vi "KalibrierInfoMessages.vi"(8 "Fehler (Eingang, kein Fehler)":errorcluster, 11 "Kalibrier Info-Cluster in":T1) -> (0 "error out":errorcluster, 3 "Kalibrier Info Messages Array":cluster{"Label.Text":string, "Wert":bool}[](array[cluster]))   [LabVIEW 2020, in "Linearisierung v2.lvlib" / "SpanEinstellungen.lvlib"]
uses:
  SpanEinstellungen.lvlib
  Kalibrier Info Cluster.ctl
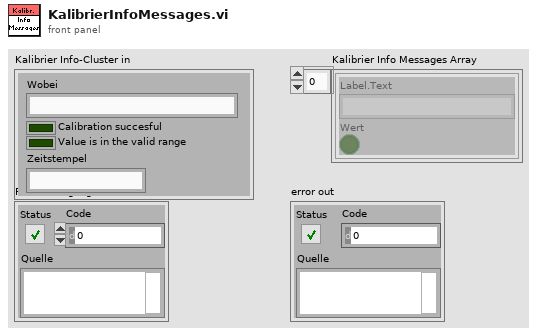
[diagram p1: front panel]
types:
  T1 = typedef "Linearisierung v2.lvlib/SpanEinstellungen.lvlib/Kalibrier Info Cluster.ctl" = cluster{"Wobei":string, "Calibration succesful":bool, "Value is in the valid range":bool, "Zeitstempel":string}
  T2 = cluster{bool, "Calibration succesful":bool, "Value is in the valid range":bool}
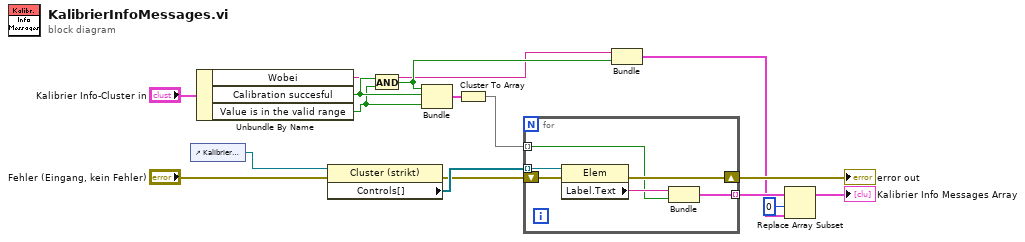
[diagram p0: block diagram]
diagram:
  n1 = control-ref of="Kalibrier Info-Cluster in"() -> (w8:refnum<vi>)
  n2 = Unbundle By Name("Kalibrier Info-Cluster in") -> ("Wobei"=w1:string, "Calibration succesful"=w7:bool, "Value is in the valid range"=w6:bool)
  n3 = property class="Cluster (strikt)"(reference=w8, error in="Fehler (Eingang, kein Fehler)") -> (error out=w14:errorcluster, "Controls[]"=w16:refnum<vi>[])  [unwired: 1 out]
  n4 = And(x=w7, y=w6) -> (x .and. y?=w3:bool)
  n5 = Bundle(w3, "Calibration succesful"=w7, "Value is in the valid range"=w6) -> (w9:T2)  [unwired: 1 in]
  n6 = Cluster To Array(cluster=w9) -> (array=w12:bool[])
  n7 = for {
    tunnel: w16 -> [w22] mode=indexing
    shift-right: [w20] -> w13
    shift-left: w14 -> [w21]
    tunnel: w12 -> [w17] mode=indexing
    tunnel: [w18] -> w11 mode=indexing
    n8 = property class="Elem"(reference=w22, error in=w21) -> (error out=w20:errorcluster, "Label.Text"=w19:string)  [unwired: 1 out]
    n9 = Bundle("Label.Text"=w19, w17) -> (w18:cluster{"Label.Text":string, bool})  [unwired: 1 in]
  }
  "error out" <- w13
  n10 = Bundle("Wobei"=w1, w3) -> (w2:cluster{"Wobei":string, bool})  [unwired: 1 in]
  n11 = Replace Array Subset(array=w11, new element=w2, index=0 ("Index")) -> (→"Kalibrier Info Messages Array":cluster{"Label.Text":string, bool}[])
